vi "PNGFile.vi"(6 "Paths error":errorcluster, 10 "PNG file path":path=path "/Users/leogallacio/Downloads/N8.png") -> (0 "Pixels colors (CLUT)":u8[](array[numeric]), 1 "Height":i16, 2 "Width":i16, 3 "Depth":i32, 4 "PNGFile error":errorcluster, 5 "Pixels colors (uchar)":u32[](array[numeric]), 7 "PNG picture":picture)   [LabVIEW 2023]
panel:
  in  "User interface":T1(tab)
  in  "User entries":enum32{""}(tab)
  in  "Customization":enum32{"Customization"}(tab)
  in  "Colors":enum32{"Colors"}(tab)
  in  "Size":enum32{"Size"}(tab)
  in  "Loop FOR 1":enum32{"Loop FOR 1"}(tab)
  in  "Arrays":enum32{"Arrays"}(tab)
  in  "Script.m":enum32{"Script.m"}(tab)
  in  "Extract.c output string scan":enum32{"Extract.c output string scan"}(tab)
  in  "T: tt1 tt2 tt3 ...":enum32{"T: tt1 tt2 tt3 ..."}(tab)
  in  "C: cc":enum32{"C: cc"}(tab)
  in  "Loop FOR 2":enum32{"Loop FOR 2"}(tab)
  in  "LabVIEW":enum32{"LabVIEW"}(tab)
  in  "MATLAB":enum32{"MATLAB"}(tab)
  in  "C":enum32{"C"}(tab)
  in  "MATLAB":enum32{"MATLAB"}(tab)
  in  "C":enum32{"C"}(tab)
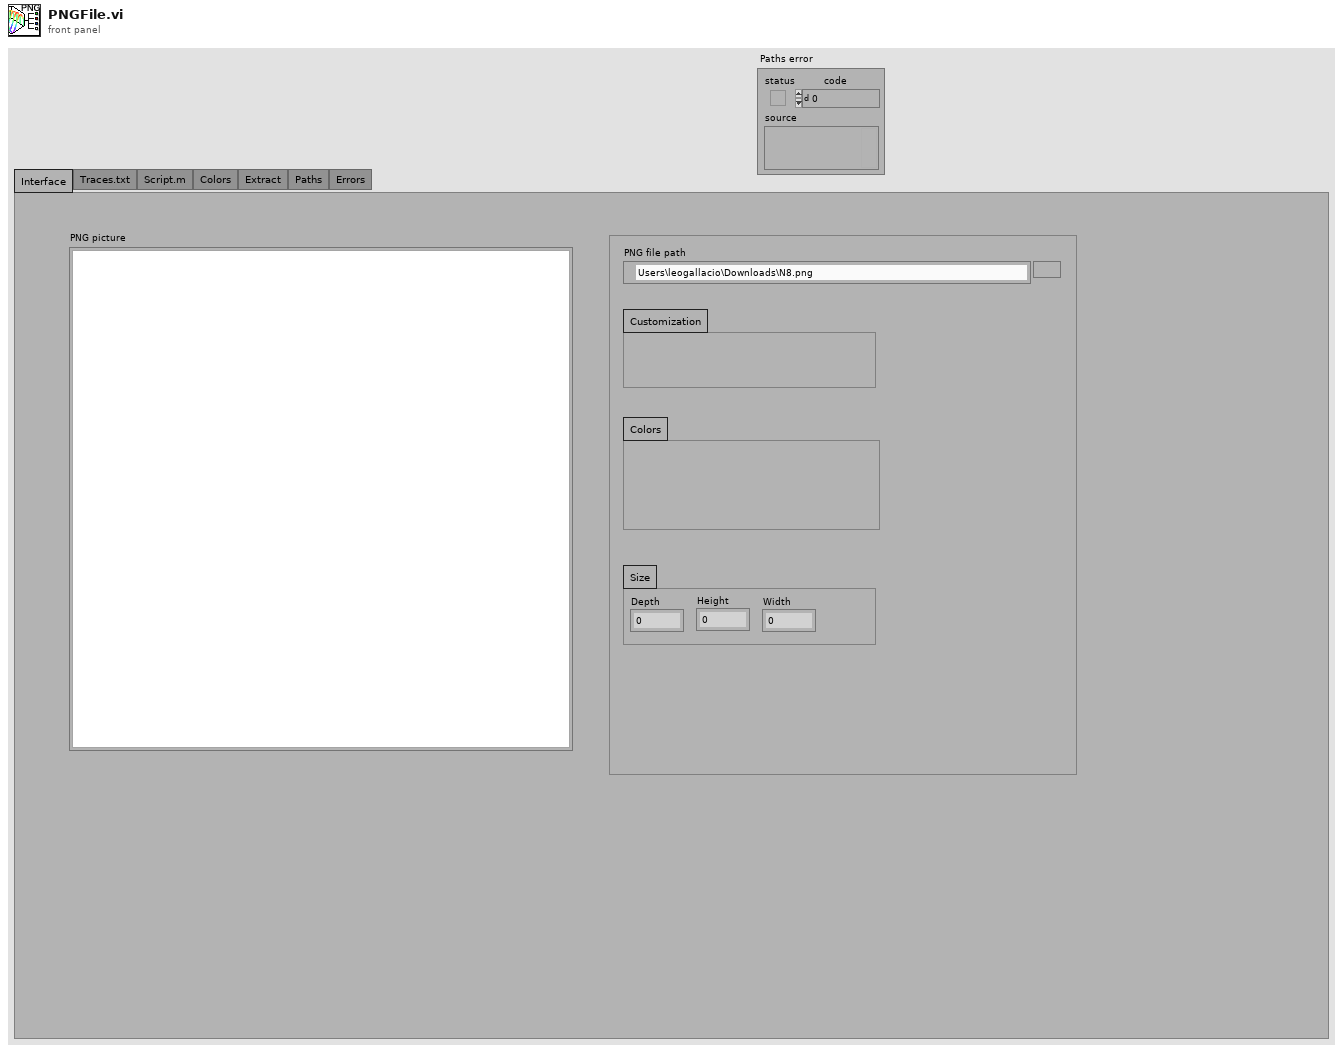
[diagram p1: front panel]
types:
  T1 = enum32{"Interface", "Traces.txt", "Script.m", "Colors", "Extract", "Paths", "Errors"}
  T2 = typedef "imagedata.ctl" = cluster{"image type":i32, "image depth":i32, "image":u8[], "mask":u8[], "colors":u32[], "Rectangle":cluster{"left":i16, "top":i16, "right":i16, "bottom":i16}}
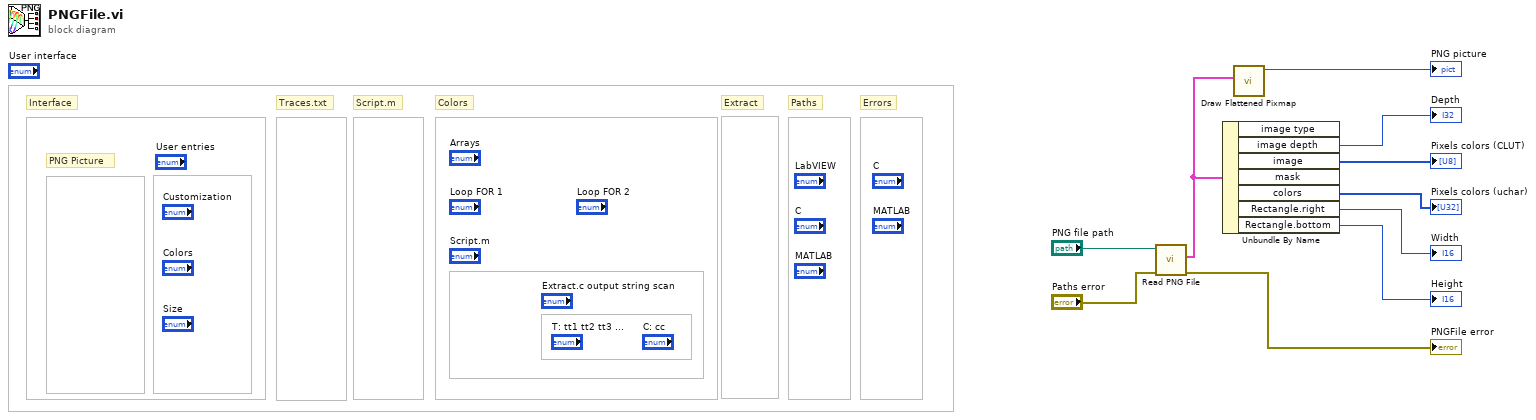
[diagram p0: block diagram]
diagram:
  # "PNG Picture"
  # "Errors"
  # "Paths"
  # "Extract"
  # "Colors"
  # "Script.m"
  # "Traces.txt"
  # "Interface"
  n1 = call <vilib>:"Read PNG File.vi"("error in (no error)"="Paths error", "path to PNG file"="PNG file path") -> ("error out"=→"PNGFile error":errorcluster, "image data"=w8:T2)  [unwired: 7 in, 1 out]
  n2 = Unbundle By Name(w8) -> ("image depth"=→"Depth":i32, "image"=→"Pixels colors (CLUT)":u8[], "colors"=→"Pixels colors (uchar)":u32[], "Rectangle.right"=→"Width":i16, "Rectangle.bottom"=→"Height":i16)  [unwired: 2 out]
  n3 = call <vilib>:"Draw Flattened Pixmap.vi"("image data"=w8) -> ("new picture"=→"PNG picture":picture)  [unwired: 8 in]
